vi "log_law.vi"(2 "z":dbl, 3 "z0":dbl, 4 "u*":dbl) -> (0 "du/dz (z)":dbl, 1 "u(z)":dbl)   [LabVIEW 2012]
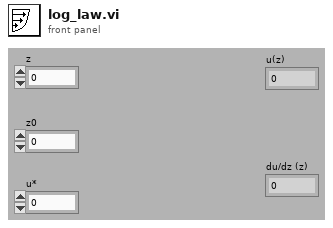
[diagram p1: front panel]
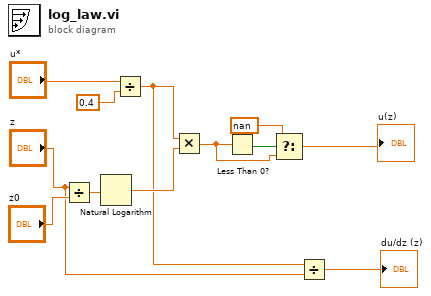
[diagram p0: block diagram]
diagram:
  n1 = Divide(x="z", y="z0") -> (x/y=w9:dbl)
  n2 = Natural Logarithm(1:w9) -> (0:w8:dbl)
  n3 = Divide(x="u*", y=0.4) -> (x/y=w3:dbl)
  n4 = Multiply(x=w3, y=w8) -> (x*y=w4:dbl)
  n5 = Less Than 0?(x=w4) -> (x < 0?=w7:bool)
  n6 = Select(t=nan, s=w7, f=w4) -> (s? t:f=→"u(z)":dbl)
  n7 = Divide(x=w3, y="z") -> (x/y=→"du/dz (z)":dbl)
